vi "KVMap-Delete.vi"(8 "T->First/F->Second(F)":bool, 10 "element":string, 11 "Cluster in":cluster{string[], string[]}) -> (3 "Cluster out":cluster{string[], string[]})   [LabVIEW 2014]
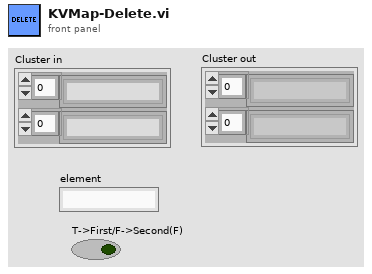
[diagram p1: front panel]
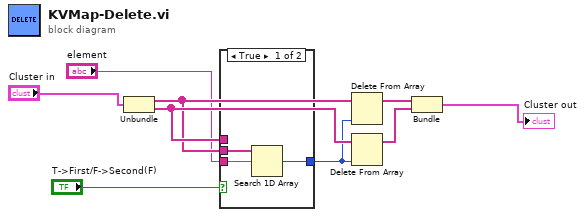
[diagram p0: block diagram]
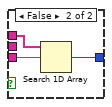
[diagram p2: hidden frame]
diagram:
  n1 = Unbundle("Cluster in") -> (w3:string[], w8:string[])
  n2 = case shown="True" "T->First/F->Second(F)" {
    tunnel: "element" -> [w12 w15]
    tunnel: w3 -> [w11 _]
    tunnel: [w10 w14] -> w4
    tunnel: w8 -> [_ w13]
    frame True {
      n3 = Search 1D Array(1D array=w11, element=w12) -> (index of element=w10:i32)  [unwired: 1 in]
    }
    frame False {
      n4 = Search 1D Array(1D array=w13, element=w15) -> (index of element=w14:i32)  [unwired: 1 in]
    }
  }
  n5 = Delete From Array(array=w3, index=w4) -> (array with subset deleted=w5:string[])  [unwired: 1 in, 1 out]
  n6 = Delete From Array(array=w8, index=w4) -> (array with subset deleted=w6:string[])  [unwired: 1 in, 1 out]
  n7 = Bundle(w5, w6) -> (→"Cluster out":cluster{string[], string[]})  [unwired: 1 in]
